vi "labVIEW_file.vi"() -> ()   [LabVIEW 2019]
uses:
  <vilib>/Instr/_visa.llb/VISA Configure Serial Port (Instr).vi
  <vilib>/Utility/file.llb/Write Delimited Spreadsheet (DBL).vi
panel:
  out "布尔":bool
  in  "file path (dialog if empty)":path=path "D:/我/学习/S3课程设计/L.xls" caption="亮度文件保存路径 （空时为对话框）"
  in  "湿度存储路径":path=path "D:/我/学习/S3课程设计/H.xls" caption="湿度文件保存路径 （空时为对话框）"
  in  "存储路径":path=path "D:/我/学习/S3课程设计/T.xls" caption="温度文件保存路径 （空时为对话框）"
  out "信道实际频率":string
  in  "希望改变的目的信道频率":string
  in  "改变信道频率":bool
  in  "采集亮度":bool
  in  "采集湿度":bool
  in  "确认要求采集":bool
  out "亮度值":dbl
  out "湿度值":dbl
  out "温度值":dbl
  in  "配置用数组，不需要动 3":dbl[](array[numeric])
  in  "亮度横坐标":dbl[](array[numeric])=[1.0, 2.0, 3.0, 4.0, 5.0, 6.0]
  out "亮度曲线":cluster{"亮度横坐标":dbl[], dbl[]}(graph)
  out "湿度曲线":cluster{"湿度横坐标":dbl[], dbl[]}(graph)
  in  "湿度横坐标":dbl[](array[numeric])=[1.0, 2.0, 3.0, 4.0, 5.0, 6.0]
  in  "配置用数组，不需要动2":dbl[](array[numeric])
  out "温度曲线":cluster{"温度横坐标":dbl[], dbl[]}(graph)
  in  "温度横坐标":dbl[](array[numeric])=[1.0, 2.0, 3.0, 4.0, 5.0, 6.0]
  in  "配置用数组，不需要动":dbl[](array[numeric])
  in  "终端3入网":bool
  in  "终端2入网":bool
  in  "终端1入网":bool
  in  "采集温度":bool
  out "3号亮度机在网状况":bool
  out "2号湿度机在网状况":bool
  out "1号温度机在网状况":bool
  in  "终端3出网":bool
  in  "终端2出网":bool
  in  "终端1出网":bool
  out "累计字符":string
  out "error out":errorcluster {"code" format="%f"}
  in  "停止 2":bool
  out "读取值":string
  # "星型无线通信系统控制面板"
  # "采集指令"
  # "出网指令"
  # "入网指令"
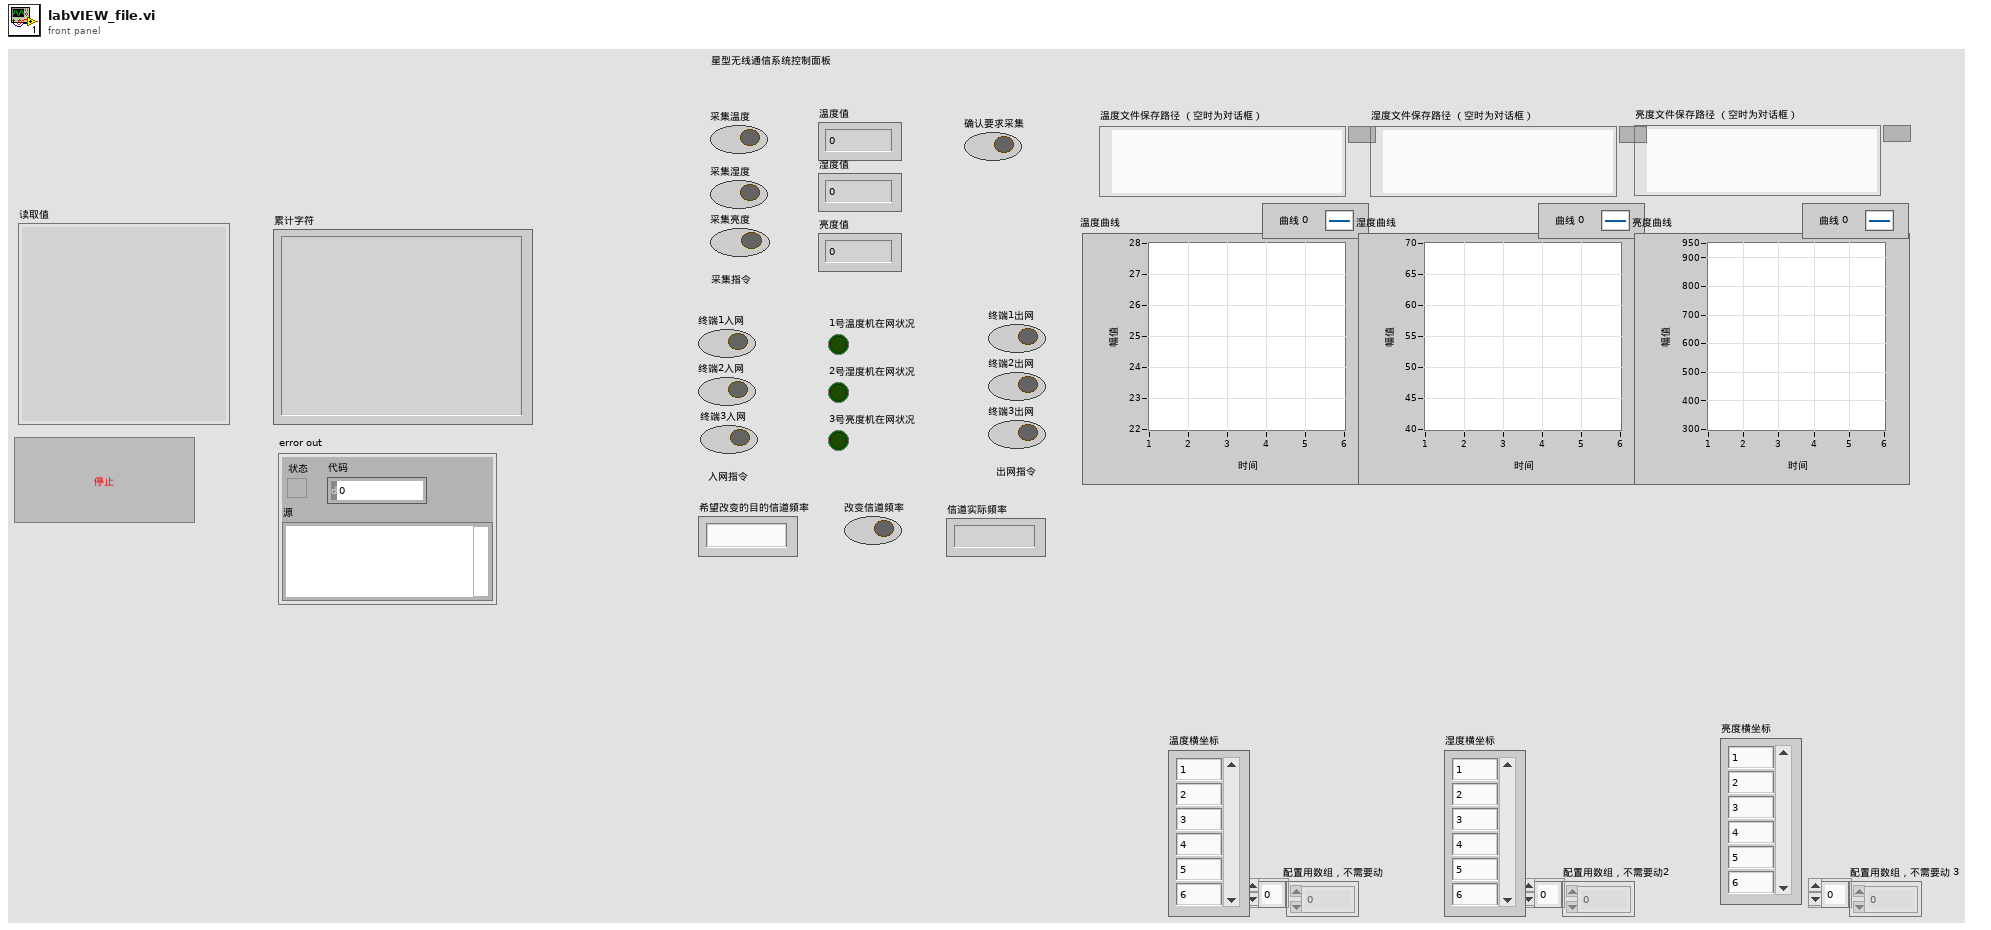
[diagram p1: front panel]
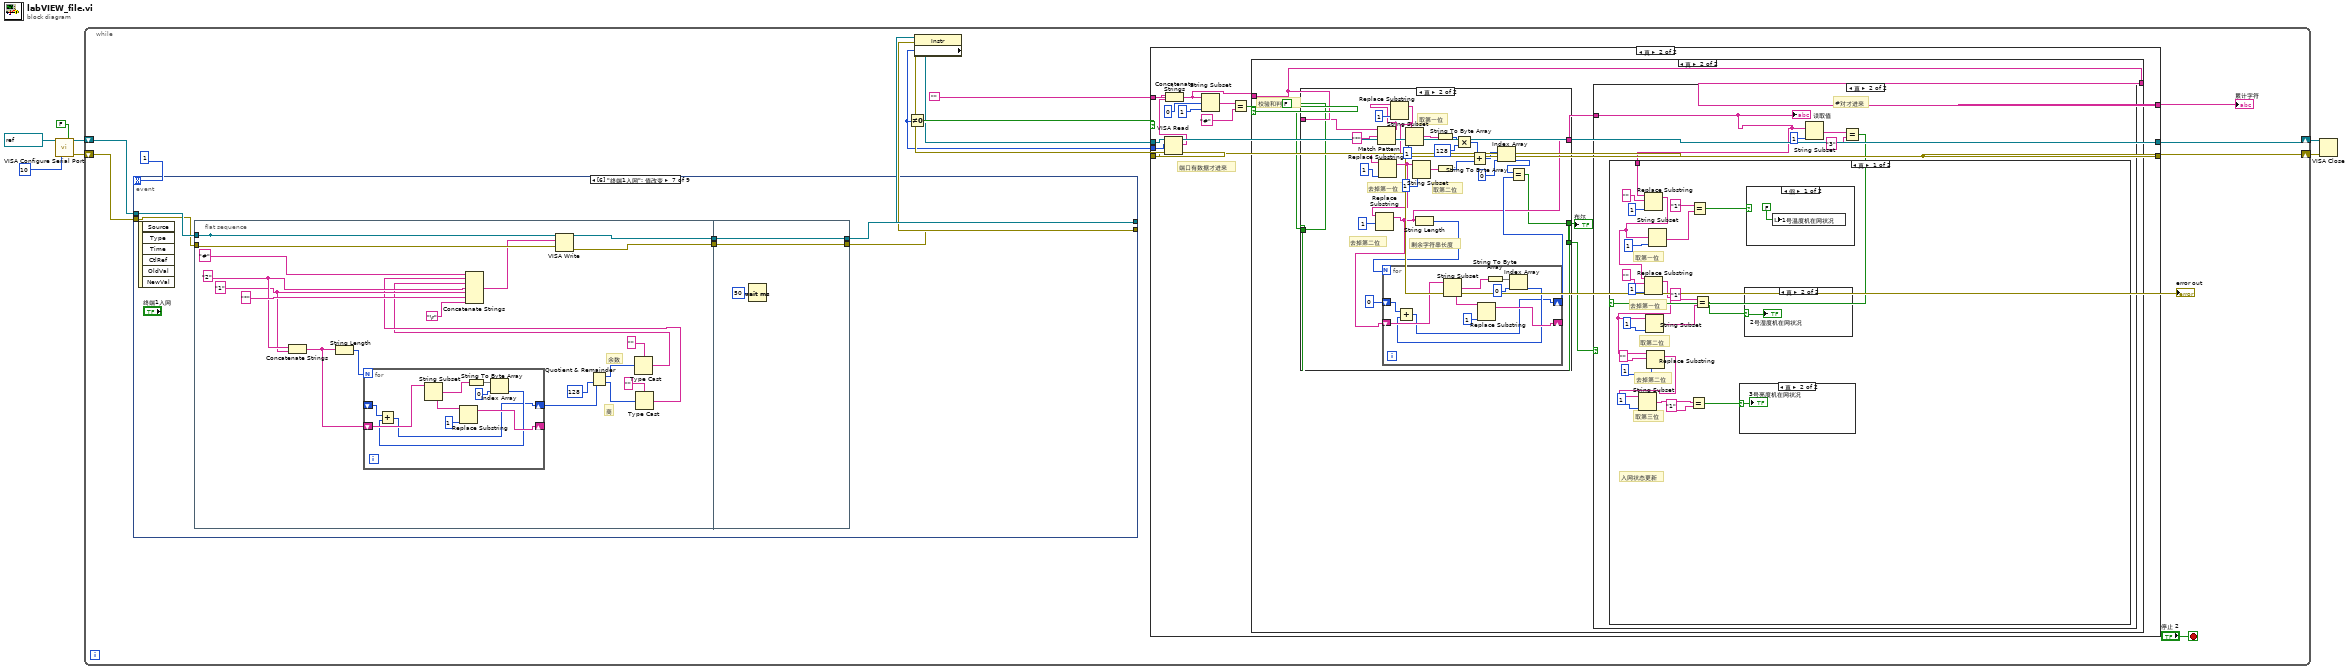
[diagram p0: block diagram]
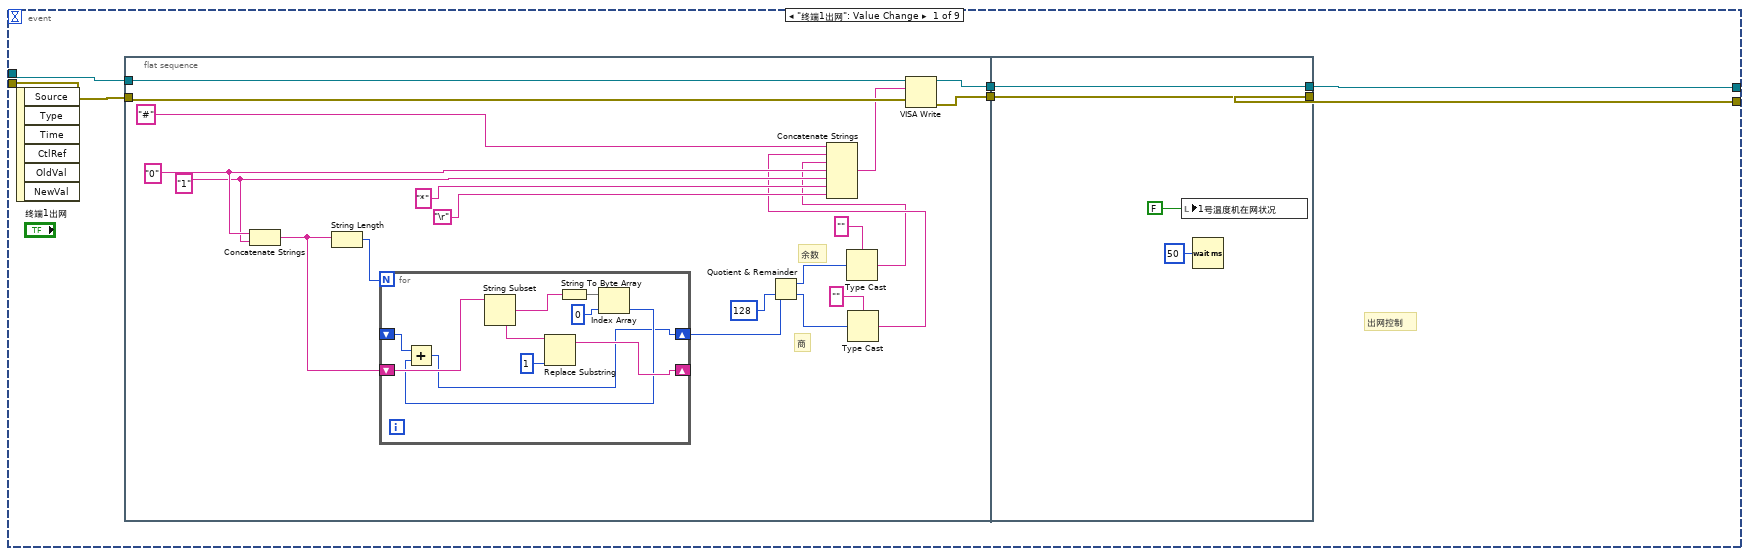
[diagram p2: hidden frame]
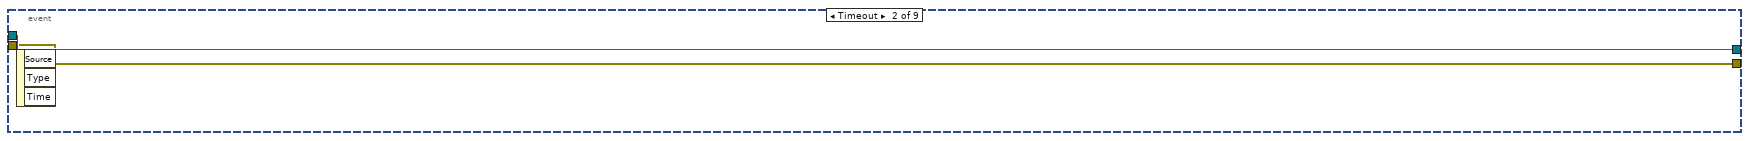
[diagram p3: hidden frame]
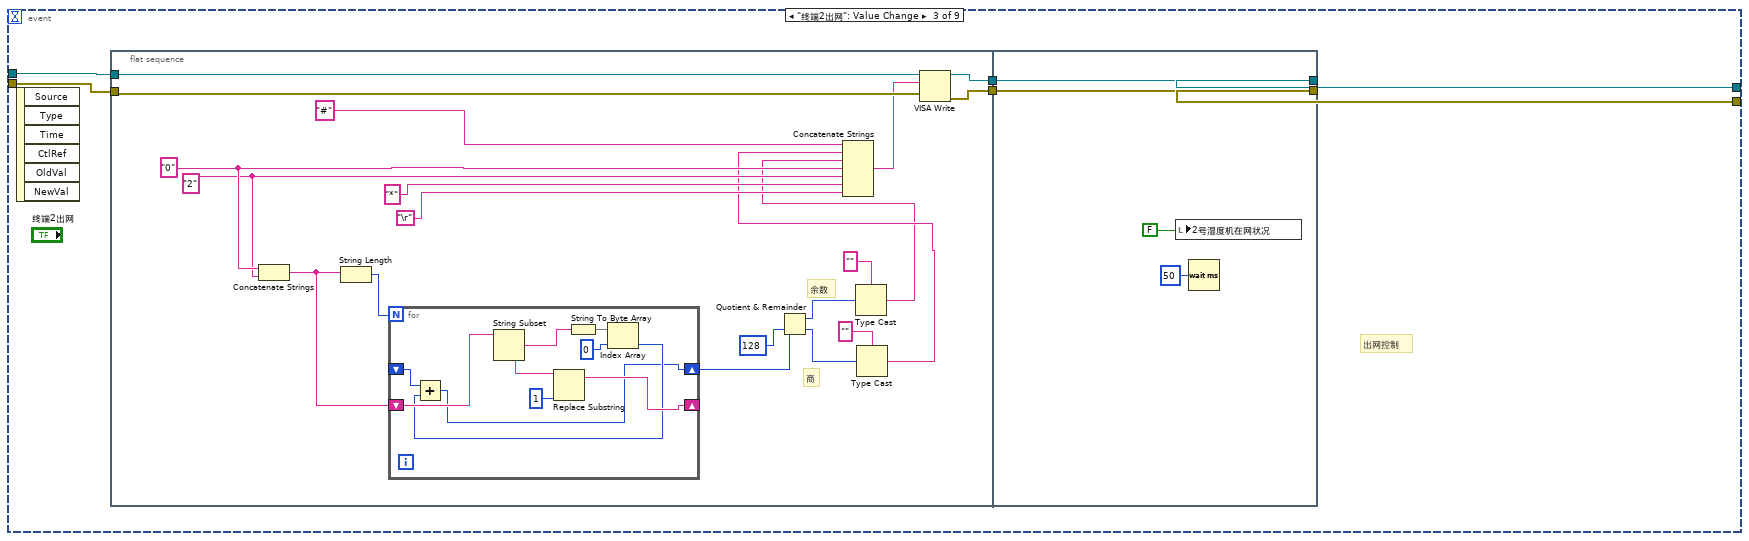
[diagram p4: hidden frame]
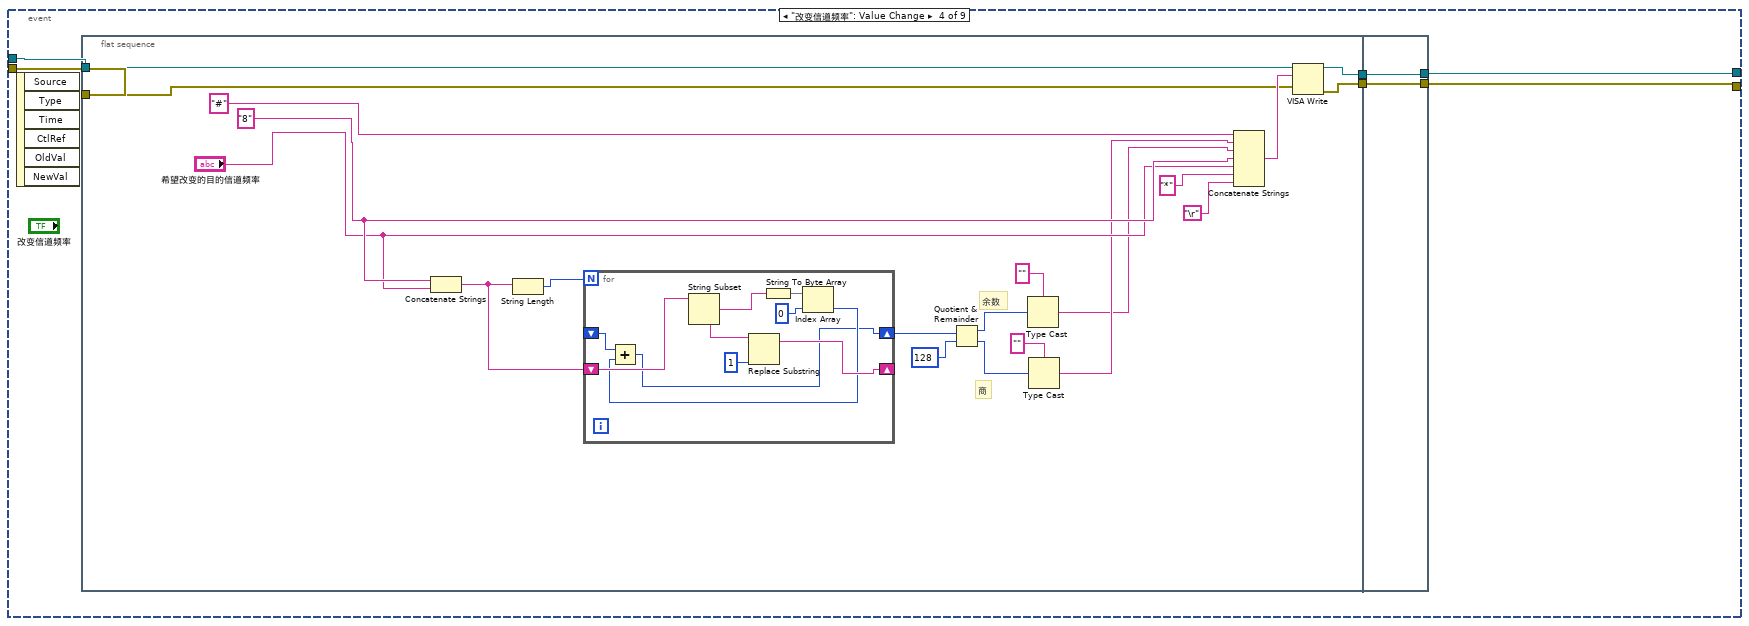
[diagram p5: hidden frame]
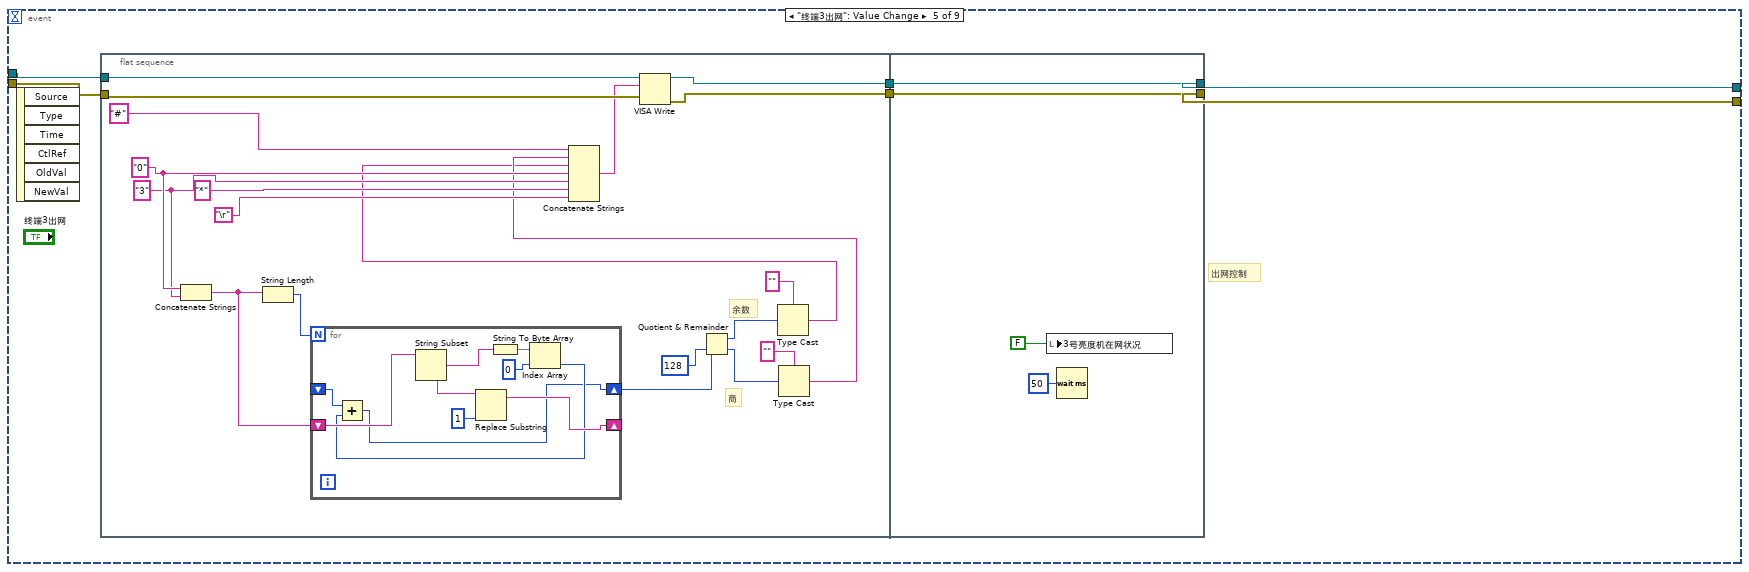
[diagram p6: hidden frame]
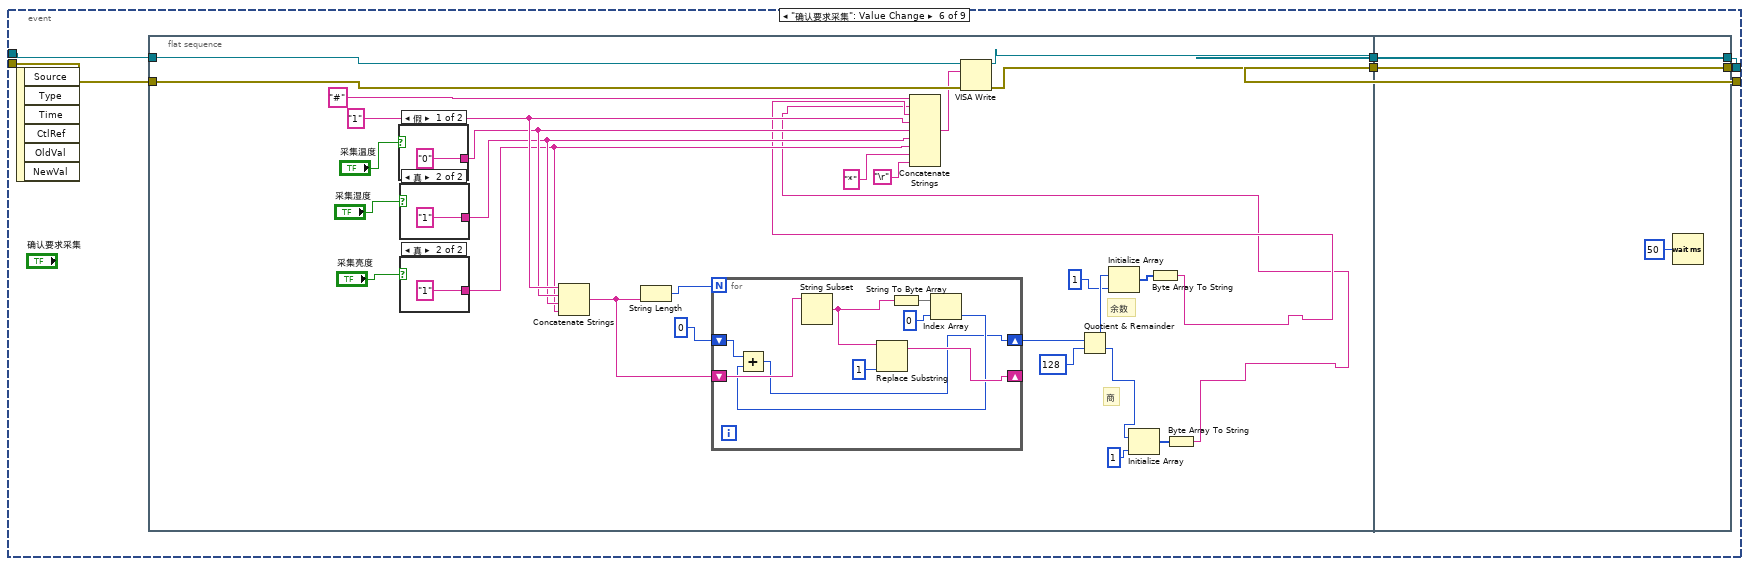
[diagram p7: hidden frame]
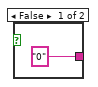
[diagram p8: hidden frame]
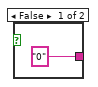
[diagram p9: hidden frame]
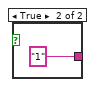
[diagram p10: hidden frame]
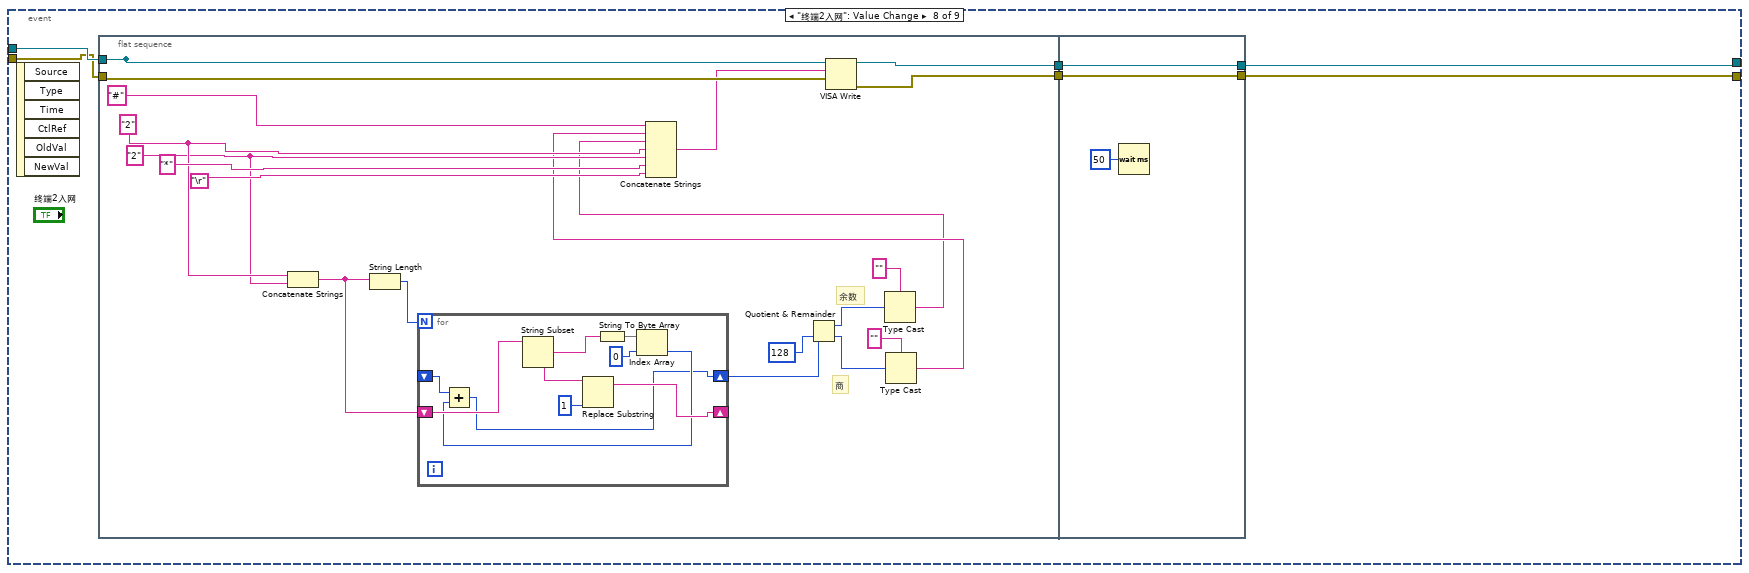
[diagram p11: hidden frame]
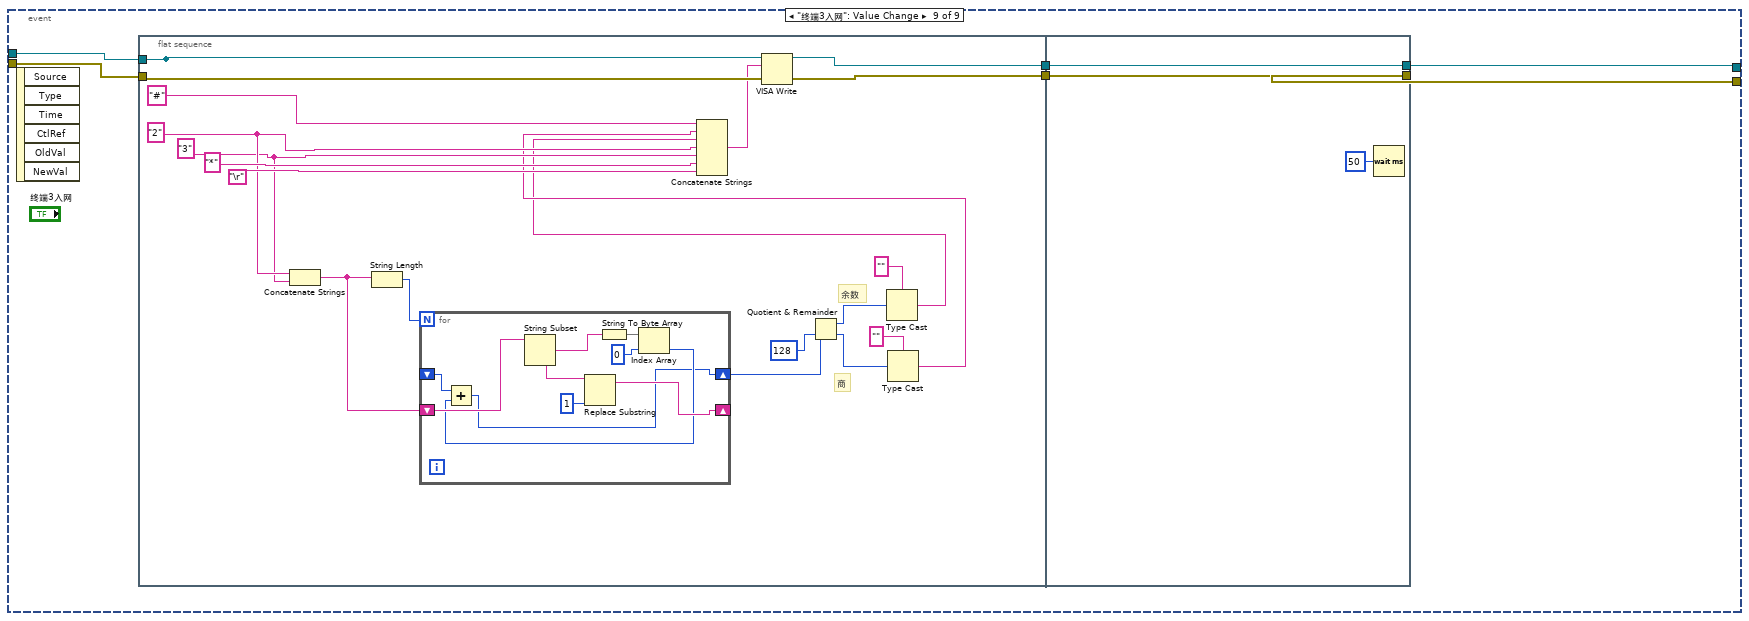
[diagram p12: hidden frame]
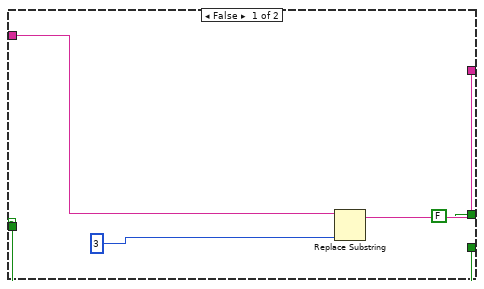
[diagram p15: hidden frame]
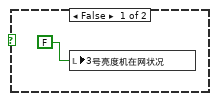
[diagram p17: hidden frame]
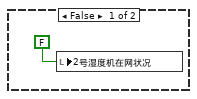
[diagram p18: hidden frame]
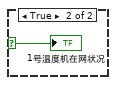
[diagram p19: hidden frame]
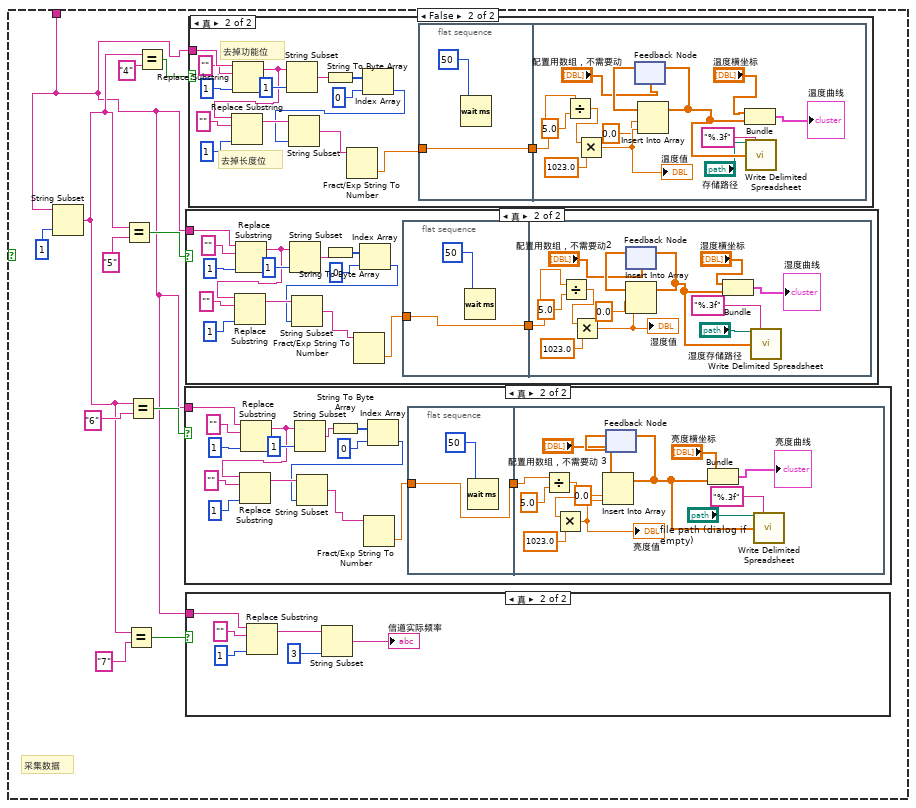
[diagram p20: hidden frame]
diagram:
  n1 = call-poly "VISA Configure Serial Port"("VISA resource name"=refnum<visa-resource-name> "COM6", "Enable Termination\nChar (T)"=FALSE ("Enable Termination\nChar (T)"), "stop bits (10: 1 bit)"=10) -> ("VISA resource name out"=w5:refnum<visa-resource-name>, "error out"=w4:errorcluster)  [unwired: 11 in]
  n2 = while {
    shift-right: [w21] -> w3
    shift-left: w5 -> [w16]
    shift-right: [w20] -> w2
    shift-left: w4 -> [w15]
    stop <- "停止 2" stop-if-true
    n3 = event shown="[6] \"终端1入网\": 值改变" {
      selector: _ -> [_ _ _ _ _ _ _ _ _]
      dyn-events: _ -> [_ _ _ _ _ _ _ _ _]
      timeout: 1 -> [_ _ _ _ _ _ _ _ _]
      tunnel: w16 -> [w27 w62 w66 w107 w142 w181 w231 w269 w309]
      tunnel: w15 -> [w26 w61 w65 w106 w141 w180 w230 w268 w308]
      tunnel: [w24 w62 w64 w104 w140 w179 w233 w271 w307] -> w13
      tunnel: [w22 w61 w63 w102 w139 w178 w232 w270 w306] -> w12
      event "终端1出网": Value Change {
        # "出网控制"
        n4 = event-data() -> ()  [unwired: 1 in, 6 out]
        n5 = flat-sequence {
          tunnel: w27 -> [w47]
          tunnel: w26 -> [w46]
          tunnel: [w44] -> w25
          tunnel: [w43] -> w23
          tunnel: [w59] -> w24
          tunnel: w25 -> [w59]
          tunnel: w23 -> [w58]
          tunnel: [w58] -> w22
          frame #0 {
            w30 = "1"
            w31 = "0"
            # "商"
            # "余数"
            n6 = Concatenate Strings(w31, w30) -> (w38:string)
            n7 = String Length(string=w38) -> (length=w39:i32)
            n8 = for {
              N: w39 -> [_]
              shift-right: [w48] -> w34
              shift-left: _ -> [w56]
              shift-right: [w50] -> _
              shift-left: w38 -> [w51]
              n9 = String Subset ("截取字符串")(string=w51) -> (substring=w55:string)  [unwired: 2 in]
              n10 = Replace Substring(2:u32 1 ("等待时间（毫秒）"), 5:w55) -> (1:w50:string)  [unwired: 2 in, 1 out]
              n11 = String To Byte Array(string=w55) -> (unsigned byte array=w53:u8[])
              n12 = Index Array(array=w53, index=u32 0 ("等待时间（毫秒）")) -> (element=w49:u8)
              n13 = Add(x=w56, y=w49) -> (x+y=w48:u8)
            }
            n14 = Quotient & Remainder(x=w34, y=u8 128 ("等待时间（毫秒）")) -> (x-y*floor(x/y)=w37:u8, floor(x/y)=w36:u8)
            n15 = Type Cast(type="", x=w37) -> (*(type *) &x=w28:string)
            n16 = Type Cast(type="", x=w36) -> (*(type *) &x=w29:string)
            n17 = Concatenate Strings("#", w29, w28, w31, w30, "*", "\r" ("回车键常量")) -> (w45:string)
            n18 = VISA Write(VISA resource name=w47, write buffer=w45, error in (no error)=w46) -> (VISA resource name out=w44:refnum<visa-resource-name>, error out=w43:errorcluster)  [unwired: 1 out]
          }
          frame #1 {
            n19 = local write "1号温度机在网状况"(FALSE) -> ()
            n20 = Wait (ms)(milliseconds to wait=u32 50 ("等待时间（毫秒）")) -> ()  [unwired: 1 out]
          }
        }
      }
      event Timeout {
        n21 = event-data() -> ()  [unwired: 1 in, 3 out]
      }
      event "终端2出网": Value Change {
        # "出网控制"
        n22 = event-data() -> ()  [unwired: 1 in, 6 out]
        n23 = flat-sequence {
          tunnel: w66 -> [w88]
          tunnel: w65 -> [w87]
          tunnel: [w85] -> w68
          tunnel: [w84] -> w67
          tunnel: [w100] -> w64
          tunnel: w68 -> [w100]
          tunnel: w67 -> [w99]
          tunnel: [w99] -> w63
          frame #0 {
            w71 = "2"
            w72 = "0"
            # "商"
            # "余数"
            n24 = Concatenate Strings(w72, w71) -> (w79:string)
            n25 = String Length(string=w79) -> (length=w80:i32)
            n26 = for {
              N: w80 -> [_]
              shift-right: [w89] -> w75
              shift-left: _ -> [w97]
              shift-right: [w91] -> _
              shift-left: w79 -> [w92]
              n27 = String Subset ("截取字符串")(string=w92) -> (substring=w96:string)  [unwired: 2 in]
              n28 = Replace Substring(2:u32 1 ("等待时间（毫秒）"), 5:w96) -> (1:w91:string)  [unwired: 2 in, 1 out]
              n29 = String To Byte Array(string=w96) -> (unsigned byte array=w94:u8[])
              n30 = Index Array(array=w94, index=u32 0 ("等待时间（毫秒）")) -> (element=w90:u8)
              n31 = Add(x=w97, y=w90) -> (x+y=w89:u8)
            }
            n32 = Quotient & Remainder(x=w75, y=u8 128 ("等待时间（毫秒）")) -> (x-y*floor(x/y)=w78:u8, floor(x/y)=w77:u8)
            n33 = Type Cast(type="", x=w78) -> (*(type *) &x=w69:string)
            n34 = Type Cast(type="", x=w77) -> (*(type *) &x=w70:string)
            n35 = Concatenate Strings("#", w70, w69, w72, w71, "*", "\r" ("回车键常量")) -> (w86:string)
            n36 = VISA Write(VISA resource name=w88, write buffer=w86, error in (no error)=w87) -> (VISA resource name out=w85:refnum<visa-resource-name>, error out=w84:errorcluster)  [unwired: 1 out]
          }
          frame #1 {
            n37 = local write "2号湿度机在网状况"(FALSE) -> ()
            n38 = Wait (ms)(milliseconds to wait=u32 50 ("等待时间（毫秒）")) -> ()  [unwired: 1 out]
          }
        }
      }
      event "改变信道频率": Value Change {
        n39 = event-data() -> ()  [unwired: 1 in, 6 out]
        n40 = flat-sequence {
          tunnel: w107 -> [w125]
          tunnel: w106 -> [w124]
          tunnel: [w123] -> w105
          tunnel: [w122] -> w103
          tunnel: w105 -> [w138]
          tunnel: [w138] -> w104
          tunnel: w103 -> [w137]
          tunnel: [w137] -> w102
          frame #0 {
            w119 = "8"
            # "商"
            # "余数"
            n41 = Concatenate Strings(w119, "希望改变的目的信道频率") -> (w116:string)
            n42 = String Length(string=w116) -> (length=w117:i32)
            n43 = for {
              N: w117 -> [_]
              shift-right: [w128] -> w112
              shift-left: _ -> [w136]
              shift-right: [w130] -> _
              shift-left: w116 -> [w131]
              n44 = String Subset ("截取字符串")(string=w131) -> (substring=w135:string)  [unwired: 2 in]
              n45 = Replace Substring(2:u32 1 ("等待时间（毫秒）"), 5:w135) -> (1:w130:string)  [unwired: 2 in, 1 out]
              n46 = String To Byte Array(string=w135) -> (unsigned byte array=w133:u8[])
              n47 = Index Array(array=w133, index=u32 0 ("等待时间（毫秒）")) -> (element=w129:u8)
              n48 = Add(x=w136, y=w129) -> (x+y=w128:u8)
            }
            n49 = Quotient & Remainder(x=w112, y=u8 128 ("等待时间（毫秒）")) -> (x-y*floor(x/y)=w115:u8, floor(x/y)=w114:u8)
            n50 = Type Cast(type="", x=w115) -> (*(type *) &x=w108:string)
            n51 = Type Cast(type="", x=w114) -> (*(type *) &x=w109:string)
            n52 = Concatenate Strings("#", w109, w108, w119, "希望改变的目的信道频率", "*", "\r" ("回车键常量")) -> (w127:string)
            n53 = VISA Write(VISA resource name=w125, write buffer=w127, error in (no error)=w124) -> (VISA resource name out=w123:refnum<visa-resource-name>, error out=w122:errorcluster)  [unwired: 1 out]
          }
          frame #1 {
          }
        }
      }
      event "终端3出网": Value Change {
        # "出网控制"
        n54 = event-data() -> ()  [unwired: 1 in, 6 out]
        n55 = flat-sequence {
          tunnel: w142 -> [w164]
          tunnel: w141 -> [w163]
          tunnel: [w161] -> w144
          tunnel: [w160] -> w143
          tunnel: [w176] -> w140
          tunnel: w144 -> [w176]
          tunnel: w143 -> [w175]
          tunnel: [w175] -> w139
          frame #0 {
            w147 = "3"
            w148 = "0"
            # "商"
            # "余数"
            n56 = Concatenate Strings(w148, w147) -> (w155:string)
            n57 = String Length(string=w155) -> (length=w156:i32)
            n58 = for {
              N: w156 -> [_]
              shift-right: [w165] -> w151
              shift-left: _ -> [w173]
              shift-right: [w167] -> _
              shift-left: w155 -> [w168]
              n59 = String Subset ("截取字符串")(string=w168) -> (substring=w172:string)  [unwired: 2 in]
              n60 = Replace Substring(2:u32 1 ("等待时间（毫秒）"), 5:w172) -> (1:w167:string)  [unwired: 2 in, 1 out]
              n61 = String To Byte Array(string=w172) -> (unsigned byte array=w170:u8[])
              n62 = Index Array(array=w170, index=u32 0 ("等待时间（毫秒）")) -> (element=w166:u8)
              n63 = Add(x=w173, y=w166) -> (x+y=w165:u8)
            }
            n64 = Quotient & Remainder(x=w151, y=u8 128 ("等待时间（毫秒）")) -> (x-y*floor(x/y)=w154:u8, floor(x/y)=w153:u8)
            n65 = Type Cast(type="", x=w154) -> (*(type *) &x=w145:string)
            n66 = Type Cast(type="", x=w153) -> (*(type *) &x=w146:string)
            n67 = Concatenate Strings("#", w146, w145, w148, w147, "*", "\r" ("回车键常量")) -> (w162:string)
            n68 = VISA Write(VISA resource name=w164, write buffer=w162, error in (no error)=w163) -> (VISA resource name out=w161:refnum<visa-resource-name>, error out=w160:errorcluster)  [unwired: 1 out]
          }
          frame #1 {
            n69 = local write "3号亮度机在网状况"(FALSE) -> ()
            n70 = Wait (ms)(milliseconds to wait=u32 50 ("等待时间（毫秒）")) -> ()  [unwired: 1 out]
          }
        }
      }
      event "确认要求采集": Value Change {
        n71 = event-data() -> ()  [unwired: 1 in, 6 out]
        n72 = flat-sequence {
          tunnel: w181 -> [w211]
          tunnel: w180 -> [w209]
          tunnel: [w210] -> w183
          tunnel: [w208] -> w182
          tunnel: [w228] -> w178
          tunnel: [w229] -> w179
          tunnel: w183 -> [w229]
          tunnel: w182 -> [w228]
          frame #0 {
            w196 = "1"
            # "商"
            # "余数"
            n73 = case shown="假" "采集温度" {
              tunnel: ["0" "1"] -> w195
              frame False {
              }
              frame True {
              }
            }
            n74 = case shown="真" "采集湿度" {
              tunnel: ["0" "1"] -> w194
              frame False {
              }
              frame True {
              }
            }
            n75 = case shown="真" "采集亮度" {
              tunnel: ["0" "1"] -> w193
              frame False {
              }
              frame True {
              }
            }
            n76 = Concatenate Strings(w196, w195, w194, w193) -> (w199:string)
            n77 = String Length(string=w199) -> (length=w200:i32)
            n78 = for {
              N: w200 -> [_]
              shift-right: [w212] -> w197
              shift-left: u32 0 ("等待时间（毫秒）") -> [w220]
              shift-right: [w214] -> _
              shift-left: w199 -> [w215]
              n79 = String Subset ("截取字符串")(string=w215) -> (substring=w219:string)  [unwired: 2 in]
              n80 = Replace Substring(2:u32 1 ("等待时间（毫秒）"), 5:w219) -> (1:w214:string)  [unwired: 2 in, 1 out]
              n81 = String To Byte Array(string=w219) -> (unsigned byte array=w217:u8[])
              n82 = Index Array(array=w217, index=u32 0 ("等待时间（毫秒）")) -> (element=w213:u8)
              n83 = Add(x=w220, y=w213) -> (x+y=w212:u32)
            }
            n84 = Quotient & Remainder(x=w197, y=u8 128 ("等待时间（毫秒）")) -> (x-y*floor(x/y)=w191:u32, floor(x/y)=w189:u32)
            n85 = Initialize Array(w191, u8 1 ("等待时间（毫秒）")) -> (w190:u32[])
            n86 = Initialize Array(w189, u8 1 ("等待时间（毫秒）")) -> (w188:u32[])
            n87 = Byte Array To String(unsigned byte array=w190) -> (string=w187:string)
            n88 = Byte Array To String(unsigned byte array=w188) -> (string=w186:string)
            n89 = Concatenate Strings("#", w186, w187, w196, w195, w194, w193, "*", "\r" ("回车键常量")) -> (w207:string)
            n90 = VISA Write(VISA resource name=w211, write buffer=w207, error in (no error)=w209) -> (VISA resource name out=w210:refnum<visa-resource-name>, error out=w208:errorcluster)  [unwired: 1 out]
          }
          frame #1 {
            n91 = Wait (ms)(milliseconds to wait=u32 50 ("等待时间（毫秒）")) -> ()  [unwired: 1 out]
          }
        }
      }
      event "终端1入网": Value Change {
        n92 = event-data() -> ()  [unwired: 1 in, 6 out]
        n93 = flat-sequence {
          tunnel: [w250] -> _
          tunnel: w230 -> [w255]
          tunnel: [w253] -> w235
          tunnel: [w252] -> w234
          tunnel: w231 -> [w250]
          tunnel: [w266] -> w233
          tunnel: w235 -> [w266]
          tunnel: w234 -> [w265]
          tunnel: [w265] -> w232
          frame #0 {
            w238 = "1"
            w239 = "2"
            # "商"
            # "余数"
            n94 = Concatenate Strings(w239, w238) -> (w246:string)
            n95 = String Length(string=w246) -> (length=w247:i32)
            n96 = for {
              N: w247 -> [_]
              shift-right: [w256] -> w242
              shift-left: _ -> [w264]
              shift-right: [w258] -> _
              shift-left: w246 -> [w259]
              n97 = String Subset ("截取字符串")(string=w259) -> (substring=w263:string)  [unwired: 2 in]
              n98 = Replace Substring(2:u32 1 ("等待时间（毫秒）"), 5:w263) -> (1:w258:string)  [unwired: 2 in, 1 out]
              n99 = String To Byte Array(string=w263) -> (unsigned byte array=w261:u8[])
              n100 = Index Array(array=w261, index=u32 0 ("等待时间（毫秒）")) -> (element=w257:u8)
              n101 = Add(x=w264, y=w257) -> (x+y=w256:u8)
            }
            n102 = Quotient & Remainder(x=w242, y=u8 128 ("等待时间（毫秒）")) -> (x-y*floor(x/y)=w245:u8, floor(x/y)=w244:u8)
            n103 = Type Cast(type="", x=w245) -> (*(type *) &x=w236:string)
            n104 = Type Cast(type="", x=w244) -> (*(type *) &x=w237:string)
            n105 = Concatenate Strings("#", w237, w236, w239, w238, "*", "\r" ("回车键常量")) -> (w254:string)
            n106 = VISA Write(VISA resource name=w250, write buffer=w254, error in (no error)=w255) -> (VISA resource name out=w253:refnum<visa-resource-name>, error out=w252:errorcluster)  [unwired: 1 out]
          }
          frame #1 {
            n107 = Wait (ms)(milliseconds to wait=u32 50 ("等待时间（毫秒）")) -> ()  [unwired: 1 out]
          }
        }
      }
      event "终端2入网": Value Change {
        n108 = event-data() -> ()  [unwired: 1 in, 6 out]
        n109 = flat-sequence {
          tunnel: w269 -> [w288]
          tunnel: w268 -> [w293]
          tunnel: [w291] -> w273
          tunnel: [w290] -> w272
          tunnel: [w288] -> _
          tunnel: [w304] -> w271
          tunnel: w273 -> [w304]
          tunnel: w272 -> [w303]
          tunnel: [w303] -> w270
          frame #0 {
            w276 = "2"
            w277 = "2"
            # "商"
            # "余数"
            n110 = Concatenate Strings(w277, w276) -> (w284:string)
            n111 = String Length(string=w284) -> (length=w285:i32)
            n112 = for {
              N: w285 -> [_]
              shift-right: [w294] -> w280
              shift-left: _ -> [w302]
              shift-right: [w296] -> _
              shift-left: w284 -> [w297]
              n113 = String Subset ("截取字符串")(string=w297) -> (substring=w301:string)  [unwired: 2 in]
              n114 = Replace Substring(2:u32 1 ("等待时间（毫秒）"), 5:w301) -> (1:w296:string)  [unwired: 2 in, 1 out]
              n115 = String To Byte Array(string=w301) -> (unsigned byte array=w299:u8[])
              n116 = Index Array(array=w299, index=u32 0 ("等待时间（毫秒）")) -> (element=w295:u8)
              n117 = Add(x=w302, y=w295) -> (x+y=w294:u8)
            }
            n118 = Quotient & Remainder(x=w280, y=u8 128 ("等待时间（毫秒）")) -> (x-y*floor(x/y)=w283:u8, floor(x/y)=w282:u8)
            n119 = Type Cast(type="", x=w283) -> (*(type *) &x=w274:string)
            n120 = Type Cast(type="", x=w282) -> (*(type *) &x=w275:string)
            n121 = Concatenate Strings("#", w275, w274, w277, w276, "*", "\r" ("回车键常量")) -> (w292:string)
            n122 = VISA Write(VISA resource name=w288, write buffer=w292, error in (no error)=w293) -> (VISA resource name out=w291:refnum<visa-resource-name>, error out=w290:errorcluster)  [unwired: 1 out]
          }
          frame #1 {
            n123 = Wait (ms)(milliseconds to wait=u32 50 ("等待时间（毫秒）")) -> ()  [unwired: 1 out]
          }
        }
      }
      event "终端3入网": Value Change {
        n124 = event-data() -> ()  [unwired: 1 in, 6 out]
        n125 = flat-sequence {
          tunnel: w309 -> [w326]
          tunnel: w308 -> [w331]
          tunnel: [w329] -> w311
          tunnel: [w328] -> w310
          tunnel: [w326] -> _
          tunnel: [w342] -> w307
          tunnel: w311 -> [w342]
          tunnel: w310 -> [w341]
          tunnel: [w341] -> w306
          frame #0 {
            w314 = "3"
            w315 = "2"
            # "商"
            # "余数"
            n126 = Concatenate Strings(w315, w314) -> (w322:string)
            n127 = String Length(string=w322) -> (length=w323:i32)
            n128 = for {
              N: w323 -> [_]
              shift-right: [w332] -> w318
              shift-left: _ -> [w340]
              shift-right: [w334] -> _
              shift-left: w322 -> [w335]
              n129 = String Subset ("截取字符串")(string=w335) -> (substring=w339:string)  [unwired: 2 in]
              n130 = Replace Substring(2:u32 1 ("等待时间（毫秒）"), 5:w339) -> (1:w334:string)  [unwired: 2 in, 1 out]
              n131 = String To Byte Array(string=w339) -> (unsigned byte array=w337:u8[])
              n132 = Index Array(array=w337, index=u32 0 ("等待时间（毫秒）")) -> (element=w333:u8)
              n133 = Add(x=w340, y=w333) -> (x+y=w332:u8)
            }
            n134 = Quotient & Remainder(x=w318, y=u8 128 ("等待时间（毫秒）")) -> (x-y*floor(x/y)=w321:u8, floor(x/y)=w320:u8)
            n135 = Type Cast(type="", x=w321) -> (*(type *) &x=w312:string)
            n136 = Type Cast(type="", x=w320) -> (*(type *) &x=w313:string)
            n137 = Concatenate Strings("#", w313, w312, w315, w314, "*", "\r" ("回车键常量")) -> (w330:string)
            n138 = VISA Write(VISA resource name=w326, write buffer=w330, error in (no error)=w331) -> (VISA resource name out=w329:refnum<visa-resource-name>, error out=w328:errorcluster)  [unwired: 1 out]
          }
          frame #1 {
            n139 = Wait (ms)(milliseconds to wait=u32 50 ("等待时间（毫秒）")) -> ()  [unwired: 1 out]
          }
        }
      }
    }
    n140 = property class="Instr"(reference=w13, error in=w12) -> (reference out=w11:refnum<visa-resource-name>, error out=w10:errorcluster, "Serial Settings:Number of Bytes at Serial Port"=w9:u32)
    n141 = Not Equal To 0?(x=w9) -> (x != 0?=w18:bool)
    n142 = case shown="真" w18 {
      tunnel: [w346 w360] -> w21
      tunnel: [w345 w359] -> w20
      tunnel: w10 -> [w345 w356]
      tunnel: w11 -> [w346 w357]
      tunnel: "" -> [w344 w358]
      tunnel: [w344 w347] -> w17
      tunnel: w9 -> [_ w355]
      frame False {
      }
      frame True {
        # "端口有数据才进来"
        n143 = VISA Read(VISA resource name=w357, byte count=w355, error in (no error)=w356) -> (VISA resource name out=w360:refnum<visa-resource-name>, read buffer=w354:string, error out=w359:errorcluster)  [unwired: 1 out]
        n144 = Concatenate Strings(w358, w354) -> (w348:string)
        n145 = String Subset ("截取字符串")(string=w348, offset (0)=u32 0 ("等待时间（毫秒）"), length (rest)=u32 1 ("等待时间（毫秒）")) -> (substring=w349:string)
        n146 = Equal?(x=w349, y="#") -> (x = y?=w350:bool)
        n147 = case shown="真" w350 {
          selector: w350 -> [_ w365]
          tunnel: w348 -> [w361 w366]
          tunnel: [w361 w366] -> w347
          frame False {
          }
          frame True {
            # "校验和判断"
            n148 = case shown="真" FALSE {
              selector: FALSE -> [_ w374]
              tunnel: [w370 w382] -> w367
              tunnel: w366 -> [w371 w375]
              tunnel: w365 -> [w369 _]
              tunnel: [w369 w374] -> w364
              tunnel: [FALSE w373] -> w362
              frame False {
                n149 = Replace Substring(2:u32 3 ("等待时间（毫秒）"), 5:w371) -> (1:w370:string)  [unwired: 2 in, 1 out]
              }
              frame True {
                # "剩余字符串长度"
                # "去掉第二位"
                # "取第二位"
                # "去掉第一位"
                # "取第一位"
                n150 = Match Pattern(string=w375, regular expression="*") -> (before substring=w378:string)  [unwired: 1 in, 3 out]
                n151 = Replace Substring(2:u32 1 ("等待时间（毫秒）"), 5:w378) -> (1:w376:string)  [unwired: 2 in, 1 out]
                n152 = Replace Substring(2:u32 1 ("等待时间（毫秒）"), 5:w376) -> (1:w390:string)  [unwired: 2 in, 1 out]
                n153 = Replace Substring(2:u32 1 ("等待时间（毫秒）"), 5:w390) -> (1:w382:string)  [unwired: 2 in, 1 out]
                n154 = String Subset ("截取字符串")(string=w376, length (rest)=u32 1 ("等待时间（毫秒）")) -> (substring=w377:string)  [unwired: 1 in]
                n155 = String Subset ("截取字符串")(string=w390, length (rest)=u32 1 ("等待时间（毫秒）")) -> (substring=w393:string)  [unwired: 1 in]
                n156 = String Length(string=w382) -> (length=w388:i32)
                n157 = for {
                  N: w388 -> [_]
                  shift-right: [w398] -> w386
                  shift-left: u32 0 ("等待时间（毫秒）") -> [w406]
                  shift-right: [w400] -> _
                  shift-left: w382 -> [w401]
                  n158 = String Subset ("截取字符串")(string=w401) -> (substring=w405:string)  [unwired: 2 in]
                  n159 = Replace Substring(2:u32 1 ("等待时间（毫秒）"), 5:w405) -> (1:w400:string)  [unwired: 2 in, 1 out]
                  n160 = String To Byte Array(string=w405) -> (unsigned byte array=w403:u8[])
                  n161 = Index Array(array=w403, index=u32 0 ("等待时间（毫秒）")) -> (element=w399:u8)
                  n162 = Add(x=w406, y=w399) -> (x+y=w398:u32)
                }
                n163 = String To Byte Array(string=w377) -> (unsigned byte array=w396:u8[])
                n164 = String To Byte Array(string=w393) -> (unsigned byte array=w392:u8[])
                n165 = Multiply(x=w396, y=u32 128 ("等待时间（毫秒）")) -> (x*y=w391:u32[])
                n166 = Add(x=w391, y=w392) -> (x+y=w385:u32[])
                n167 = Index Array(array=w385, index=u32 0 ("等待时间（毫秒）")) -> (element=w383:u32)
                n168 = Equal?(x=w383, y=w386) -> (x = y?=w373:bool)
              }
            }
            "布尔" <- w362
            n169 = case shown="真" w364 {
              tunnel: w367 -> [_ w407]
              frame False {
              }
              frame True {
                # "#对才进来"
                n170 = String Subset ("截取字符串")(string=w407, length (rest)=u32 1 ("等待时间（毫秒）")) -> (substring=w408:string)  [unwired: 1 in]
                n171 = Equal?(x=w408, y="3") -> (x = y?=w409:bool)
                n172 = case shown="真" w409 {
                  tunnel: w407 -> [w430 w440]
                  frame True {
                    # "取第三位"
                    # "去掉第二位"
                    # "取第二位"
                    # "去掉第一位"
                    # "取第一位"
                    # "入网状态更新"
                    n173 = Replace Substring(2:u32 1 ("等待时间（毫秒）"), 4:"", 5:w430) -> (1:w420:string)  [unwired: 1 in, 1 out]
                    n174 = Replace Substring(2:u32 1 ("等待时间（毫秒）"), 4:"", 5:w420) -> (1:w417:string)  [unwired: 1 in, 1 out]
                    n175 = String Subset ("截取字符串")(string=w417, length (rest)=u32 1 ("等待时间（毫秒）")) -> (substring=w418:string)  [unwired: 1 in]
                    n176 = Replace Substring(2:u32 1 ("等待时间（毫秒）"), 4:"", 5:w417) -> (1:w414:string)  [unwired: 1 in, 1 out]
                    n177 = String Subset ("截取字符串")(string=w414, length (rest)=u32 1 ("等待时间（毫秒）")) -> (substring=w412:string)  [unwired: 1 in]
                    n178 = String Subset ("截取字符串")(string=w420, length (rest)=u32 1 ("等待时间（毫秒）")) -> (substring=w429:string)  [unwired: 1 in]
                    n179 = Equal?(x=w412, y="1") -> (x = y?=w423:bool)
                    n180 = Equal?(x="1", y=w429) -> (x = y?=w425:bool)
                    n181 = Equal?(x="1", y=w418) -> (x = y?=w424:bool)
                    n182 = case shown="真" w423 {
                      selector: w423 -> [_ w435]
                      frame False {
                        n183 = local write "3号亮度机在网状况"(FALSE) -> ()
                      }
                      frame True {
                        "3号亮度机在网状况" <- w435
                      }
                    }
                    n184 = case shown="真" w424 {
                      selector: w424 -> [_ w437]
                      frame False {
                        n185 = local write "2号湿度机在网状况"(FALSE) -> ()
                      }
                      frame True {
                        "2号湿度机在网状况" <- w437
                      }
                    }
                    n186 = case shown="假" w425 {
                      selector: w425 -> [_ w439]
                      frame False {
                        n187 = local write "1号温度机在网状况"(FALSE) -> ()
                      }
                      frame True {
                        "1号温度机在网状况" <- w439
                      }
                    }
                  }
                  frame False {
                    # "采集数据"
                    n188 = String Subset ("截取字符串")(string=w440, length (rest)=u32 1 ("等待时间（毫秒）")) -> (substring=w441:string)  [unwired: 1 in]
                    n189 = Equal?(x=w441, y="5") -> (x = y?=w447:bool)
                    n190 = Equal?(x=w441, y="7") -> (x = y?=w443:bool)
                    n191 = Equal?(x=w441, y="6") -> (x = y?=w445:bool)
                    n192 = Equal?(x=w441, y="4") -> (x = y?=w449:bool)
                    n193 = case shown="真" w445 {
                      tunnel: w440 -> [_ w464]
                      frame False {
                      }
                      frame True {
                        n194 = Replace Substring(2:u32 1 ("等待时间（毫秒）"), 4:"", 5:w464) -> (1:w468:string)  [unwired: 1 in, 1 out]
                        n195 = Replace Substring(2:u32 1 ("等待时间（毫秒）"), 4:"", 5:w468) -> (1:w467:string)  [unwired: 1 in, 1 out]
                        n196 = String Subset ("截取字符串")(string=w468, length (rest)=u32 1 ("等待时间（毫秒）")) -> (substring=w461:string)  [unwired: 1 in]
                        n197 = String To Byte Array(string=w461) -> (unsigned byte array=w463:u8[])
                        n198 = Index Array(array=w463, index=u32 0 ("等待时间（毫秒）")) -> (element=w460:u8)
                        n199 = String Subset ("截取字符串")(string=w467, length (rest)=w460) -> (substring=w458:string)  [unwired: 1 in]
                        n200 = Fract/Exp String To Number(string=w458) -> (number=w457:dbl)  [unwired: 3 in, 1 out]
                        n201 = flat-sequence {
                          tunnel: w457 -> [w472]
                          tunnel: [w472] -> w459
                          tunnel: w459 -> [w479]
                          frame #0 {
                            n202 = Wait (ms)(milliseconds to wait=50) -> ()  [unwired: 1 out]
                          }
                          frame #1 {
                            n203 = Divide(x=w479, y=5.0 ("等待时间（毫秒）")) -> (x/y=w481:dbl)
                            n204 = Multiply(x=w481, y=1023.0 ("等待时间（毫秒）")) -> (x*y=w478:dbl)
                            "亮度值" <- w478
                            n205 = feedback #1("配置用数组，不需要动 3") -> (w486:dbl[])
                            n206 = Insert Into Array(array=w486, index=0.0 ("等待时间（毫秒）"), new element=w478) -> (w476:dbl[])
                            n207 = feedback-in #1(w476) -> ()
                            n208 = Bundle("亮度横坐标"="亮度横坐标", "配置用数组，不需要动 3"=w476) -> (→"亮度曲线":cluster{"亮度横坐标":dbl[], "配置用数组，不需要动 3":dbl[]})  [unwired: 1 in]
                            n209 = call-poly <vilib>:"Write Delimited Spreadsheet.vi"("file path (dialog if empty)"="file path (dialog if empty)", "format (%.3f)"="%.3f", "1D data"=w476) -> ()  [unwired: 11 in, 2 out]
                          }
                        }
                      }
                    }
                    n210 = case shown="真" w447 {
                      tunnel: w440 -> [_ w494]
                      frame False {
                      }
                      frame True {
                        n211 = Replace Substring(2:u32 1 ("等待时间（毫秒）"), 4:"", 5:w494) -> (1:w498:string)  [unwired: 1 in, 1 out]
                        n212 = Replace Substring(2:u32 1 ("等待时间（毫秒）"), 4:"", 5:w498) -> (1:w497:string)  [unwired: 1 in, 1 out]
                        n213 = String Subset ("截取字符串")(string=w498, length (rest)=u32 1 ("等待时间（毫秒）")) -> (substring=w491:string)  [unwired: 1 in]
                        n214 = String To Byte Array(string=w491) -> (unsigned byte array=w493:u8[])
                        n215 = Index Array(array=w493, index=u32 0 ("等待时间（毫秒）")) -> (element=w490:u8)
                        n216 = String Subset ("截取字符串")(string=w497, length (rest)=w490) -> (substring=w488:string)  [unwired: 1 in]
                        n217 = Fract/Exp String To Number(string=w488) -> (number=w487:dbl)  [unwired: 3 in, 1 out]
                        n218 = flat-sequence {
                          tunnel: [w502] -> w489
                          tunnel: w487 -> [w502]
                          tunnel: w489 -> [w509]
                          frame #0 {
                            n219 = Wait (ms)(milliseconds to wait=50) -> ()  [unwired: 1 out]
                          }
                          frame #1 {
                            n220 = Divide(x=w509, y=5.0 ("等待时间（毫秒）")) -> (x/y=w511:dbl)
                            n221 = Multiply(x=w511, y=1023.0 ("等待时间（毫秒）")) -> (x*y=w508:dbl)
                            "湿度值" <- w508
                            n222 = feedback #2("配置用数组，不需要动2") -> (w516:dbl[])
                            n223 = Insert Into Array(array=w516, index=0.0 ("等待时间（毫秒）"), new element=w508) -> (w506:dbl[])
                            n224 = feedback-in #2(w506) -> ()
                            n225 = Bundle("湿度横坐标"="湿度横坐标", "配置用数组，不需要动2"=w506) -> (→"湿度曲线":cluster{"湿度横坐标":dbl[], "配置用数组，不需要动2":dbl[]})  [unwired: 1 in]
                            n226 = call-poly <vilib>:"Write Delimited Spreadsheet.vi"("file path (dialog if empty)"="湿度存储路径", "format (%.3f)"="%.3f", "1D data"=w506) -> ()  [unwired: 11 in, 2 out]
                          }
                        }
                      }
                    }
                    n227 = case shown="真" w443 {
                      tunnel: w440 -> [_ w454]
                      frame False {
                      }
                      frame True {
                        n228 = Replace Substring(2:u32 1 ("等待时间（毫秒）"), 4:"", 5:w454) -> (1:w452:string)  [unwired: 1 in, 1 out]
                        n229 = String Subset ("截取字符串")(string=w452, length (rest)=u32 3 ("等待时间（毫秒）")) -> (substring=→"信道实际频率":string)  [unwired: 1 in]
                      }
                    }
                    n230 = case shown="真" w449 {
                      tunnel: w440 -> [_ w531]
                      frame False {
                      }
                      frame True {
                        # "去掉长度位"
                        # "去掉功能位"
                        n231 = Replace Substring(2:u32 1 ("等待时间（毫秒）"), 4:"", 5:w531) -> (1:w527:string)  [unwired: 1 in, 1 out]
                        n232 = Replace Substring(2:u32 1 ("等待时间（毫秒）"), 4:"", 5:w527) -> (1:w526:string)  [unwired: 1 in, 1 out]
                        n233 = String Subset ("截取字符串")(string=w527, length (rest)=u32 1 ("等待时间（毫秒）")) -> (substring=w523:string)  [unwired: 1 in]
                        n234 = String To Byte Array(string=w523) -> (unsigned byte array=w522:u8[])
                        n235 = Index Array(array=w522, index=u32 0 ("等待时间（毫秒）")) -> (element=w520:u8)
                        n236 = String Subset ("截取字符串")(string=w526, length (rest)=w520) -> (substring=w518:string)  [unwired: 1 in]
                        n237 = Fract/Exp String To Number(string=w518) -> (number=w517:dbl)  [unwired: 3 in, 1 out]
                        n238 = flat-sequence {
                          tunnel: w517 -> [w532]
                          tunnel: [w532] -> w519
                          tunnel: w519 -> [w539]
                          frame #0 {
                            n239 = Wait (ms)(milliseconds to wait=50) -> ()  [unwired: 1 out]
                          }
                          frame #1 {
                            n240 = Divide(x=w539, y=5.0 ("等待时间（毫秒）")) -> (x/y=w541:dbl)
                            n241 = Multiply(x=w541, y=1023.0 ("等待时间（毫秒）")) -> (x*y=w538:dbl)
                            "温度值" <- w538
                            n242 = feedback #3("配置用数组，不需要动") -> (w546:dbl[])
                            n243 = Insert Into Array(array=w546, index=0.0 ("等待时间（毫秒）"), new element=w538) -> (w536:dbl[])
                            n244 = feedback-in #3(w536) -> ()
                            n245 = Bundle("温度横坐标"="温度横坐标", "配置用数组，不需要动"=w536) -> (→"温度曲线":cluster{"温度横坐标":dbl[], "配置用数组，不需要动":dbl[]})  [unwired: 1 in]
                            n246 = call-poly <vilib>:"Write Delimited Spreadsheet.vi"("file path (dialog if empty)"="存储路径", "format (%.3f)"="%.3f", "1D data"=w536) -> ()  [unwired: 11 in, 2 out]
                          }
                        }
                      }
                    }
                  }
                }
                "读取值" <- w407
              }
            }
          }
        }
      }
    }
    "error out" <- w20
    "累计字符" <- w17
  }
  n247 = VISA Close(VISA resource name=w3, error in (no error)=w2) -> ()  [unwired: 1 out]
